vi "octave_command.vi"(5 "recieve interval [ms]":i32=100, 7 "timeout [ms]":i32=1000, 8 "error in":errorcluster, 9 "read buffer size (4096)":i32=4096, 10 "write buffer":string, 11 "instance handle in":u32[](array[numeric])) -> (0 "error out":errorcluster, 1 "bytes read":i32, 2 "read buffer":string, 3 "instance handle out":u32[](array[numeric]), 4 "exited":bool)   [LabVIEW 2011]
doc: "Flushes unread Octave stdout data, sends command to Octave if some specified, waits for response. Response has two timeouts: first one is first response byte timeout, second one defines maximum interval between successive response data blocks.\nIf no process instance handle is connected, last one from global variable is used or new instance handle is stored to it."
uses:
  octave_var.vi
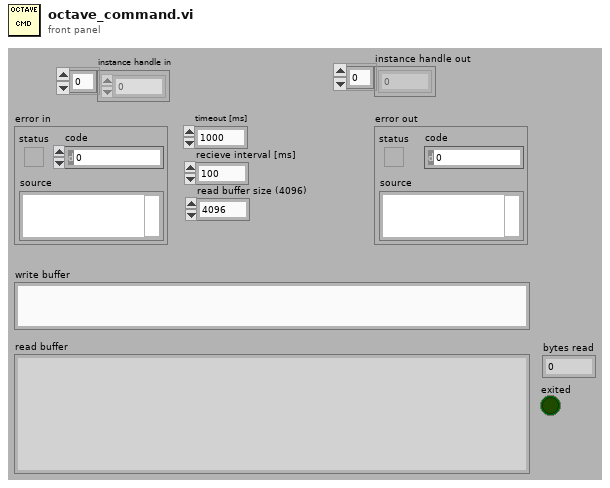
[diagram p1: front panel]
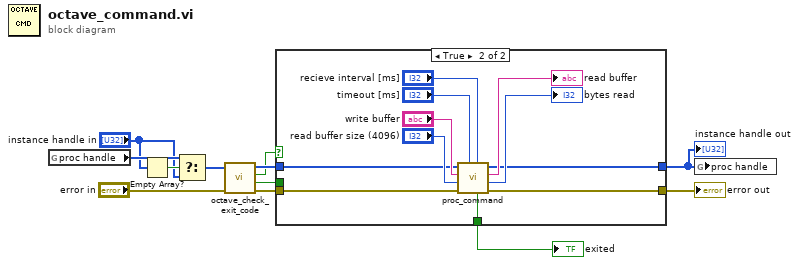
[diagram p0: block diagram]
diagram:
  n1 = global read "octave_var.vi" "proc handle"() -> (w10:u32[])
  n2 = Empty Array?(array="instance handle in") -> (empty?=w9:bool)
  n3 = Select(t=w10, s=w9, f="instance handle in") -> (s? t:f=w4:u32[])
  n4 = call "octave_check_exit_code.vi"("error in"="error in", "instance handle in"=w4) -> ("error out"=w6:errorcluster, "exited"=w1:bool, "running"=w2:bool, "instance handle out"=w3:u32[])  [unwired: 5 in, 1 out]
  n5 = case shown="True" w2 {
    tunnel: [w15 w17] -> w12
    tunnel: [w13 w20] -> w11
    tunnel: [w14 w16] -> w7
    tunnel: w6 -> [w15 w19]
    tunnel: w3 -> [w14 w18]
    tunnel: w1 -> [w13 _]
    frame False {
    }
    frame True {
      n6 = call "proc_command.vi"("recieve interval [ms]"="recieve interval [ms]", "timeout [ms]"="timeout [ms]", "error in"=w19, "read buffer size"="read buffer size (4096)", "write buffer"="write buffer", "process instance handle in"=w18) -> ("error out"=w17:errorcluster, "bytes read"=→"bytes read":i32, "read buffer"=→"read buffer":string, "process instance handle out"=w16:u32[], "exited"=w20:bool)  [unwired: 1 in]
    }
  }
  "error out" <- w12
  "exited" <- w11
  "instance handle out" <- w7
  n7 = global write "octave_var.vi" "proc handle"(w7) -> ()
